vi "Exemple_Model_Selection_LeaveOneGroupOut.vi"() -> ()   [LabVIEW 2020]
panel:
  out "Split":T1(array[cluster])
  out "error out":errorcluster caption="sortie d'erreur"
  in  "error in (no error)":errorcluster caption="entrée d'erreur (pas d'erreur)"
  in  "Groups":string[][](array[string])=[["1"], ["1"], ["2"], ["2"]]
  in  "y":string[][](array[string])=[["1"], ["2"], ["1"], ["2"]]
  in  "X":string[][](array[string])=[["1", "2"], ["3", "4"], ["5", "6"], ["7", "8"]]
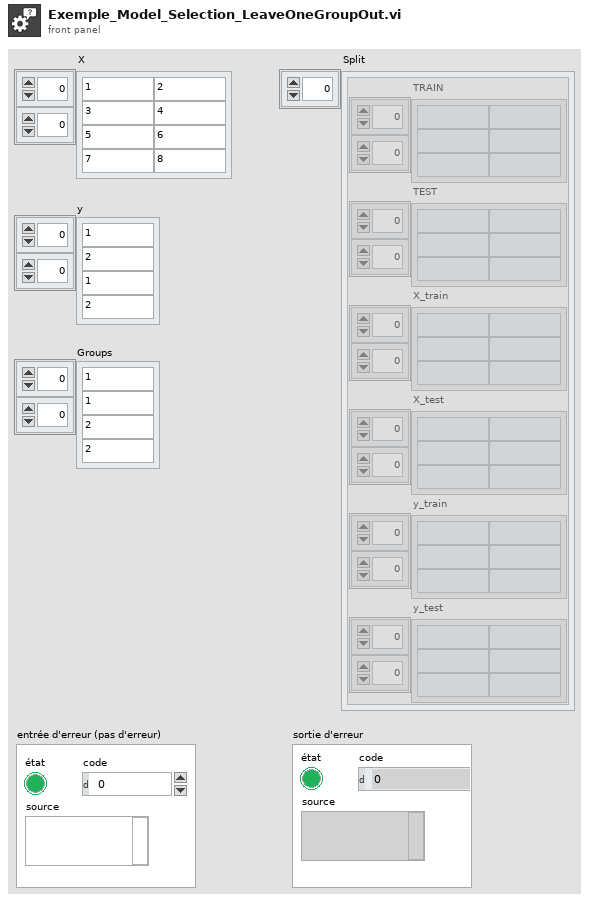
[diagram p1: front panel]
types:
  T1 = cluster{"TRAIN":string[][], "TEST":string[][], "X_train":string[][], "X_test":string[][], "y_train":string[][], "y_test":string[][]}[]
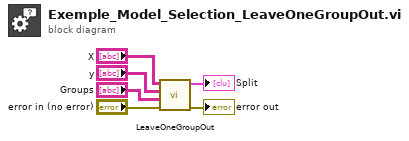
[diagram p0: block diagram]
diagram:
  n1 = call "LeaveOneGroupOut.vi"("error in (no error)"="error in (no error)", "Groups"="Groups", "y"="y", "X"="X") -> ("error out"=→"error out":errorcluster, "Split"=→"Split":T1)  [unwired: 6 in]
